vi "ULx Read (Digital 2D U8 NChan NSamp).vi"(0 "task in":refnum<k24>, 7 "number of samples per channel":i32=-1, 9 "timeout":dbl=10.0 format="%_4g", 11 "error in":errorcluster) -> (4 "task out":refnum<k24>, 6 "data":u8[][](array[numeric]), 15 "error out":errorcluster)   [LabVIEW 2020]
doc: "Reads one or more 8-bit unsigned integer samples from a task that contains one or more digital input channels. Use an instance that reads 8-bit unsigned integers for devices with up to eight lines per port."
uses:
  C:/Users/William/Documents/LV 2020 builds/LeaktestDAQ/Source-v33/ULx_LV.dll
  ULx_LV.dll
panel:
  # "sample #"
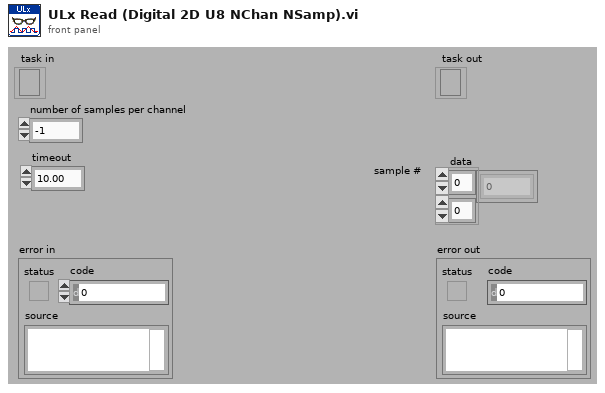
[diagram p1: front panel]
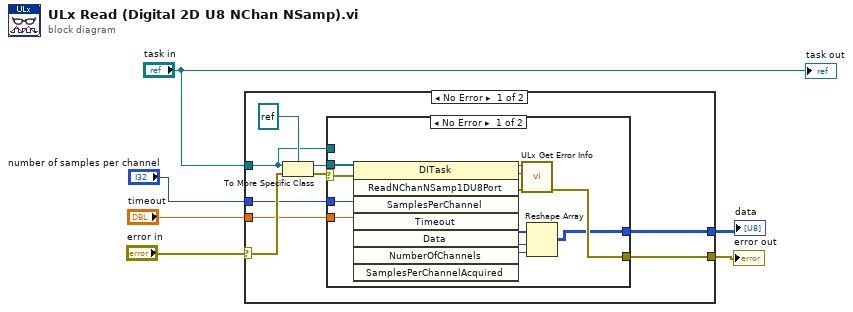
[diagram p0: block diagram]
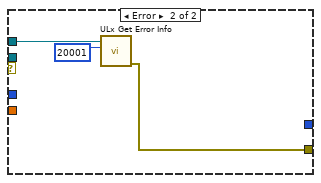
[diagram p2: hidden frame]
diagram:
  n1 = case shown="No Error" "error in" {
    selector: "error in" -> [w15 w31]
    tunnel: "task in" -> [w7 _]
    tunnel: "timeout" -> [w11 _]
    tunnel: [w10 w31] -> w4
    tunnel: "number of samples per channel" -> [w9 _]
    tunnel: [w8 _] -> w1
    frame No Error {
      n2 = To More Specific Class(target class=refnum<k24> refnum, reference=w7, error in=w15) -> (specific class reference=w12:refnum<k24>, error out=w13:errorcluster)
      n3 = case shown="No Error" w13 {
        selector: w13 -> [w26 _]
        tunnel: w12 -> [w27 _]
        tunnel: w11 -> [w22 _]
        tunnel: [w23 w28] -> w10
        tunnel: w9 -> [w21 _]
        tunnel: [w16 _] -> w8
        tunnel: w7 -> [_ w30]
        frame No Error {
          n4 = invoke class="DITask" method="ReadNChanNSamp1DU8Port"(reference=w27, error in=w26, "SamplesPerChannel"=w21, "Timeout"=w22) -> (reference out=w24:refnum<k24>, error out=w25:errorcluster, "ReadNChanNSamp1DU8Port"=w20:i32, "Data"=w18:u8[], "NumberOfChannels"=w19:i32, "SamplesPerChannelAcquired"=w17:i32)  [unwired: 4 in, 2 out]
          n5 = call "ULx Get Error Info.vi"("error in"=w25, "ErrorCode"=w20, "task in"=w24) -> ("error out"=w23:errorcluster)  [unwired: 8 in]
          n6 = Reshape Array(w18, w19, w17) -> (w16:u8[][])
        }
        frame Error {
          n7 = call "ULx Get Error Info.vi"("ErrorCode"=20001, "task in"=w30) -> ("error out"=w28:errorcluster)  [unwired: 9 in]
        }
      }
    }
    frame Error {
    }
  }
  "error out" <- w4
  "data" <- w1
  "task out" <- "task in"
